vi "Set Hidden.vi"(8 "error in (no error)":errorcluster, 11 "Panel in":refnum<class "Panel.lvclass">) -> (0 "error out":errorcluster, 3 "Panel out":refnum<class "Panel.lvclass">)   [LabVIEW 2018, in "OOPanel.lvlib" / "Panel.lvclass"]
uses:
  Panel.lvclass
  State.ctl
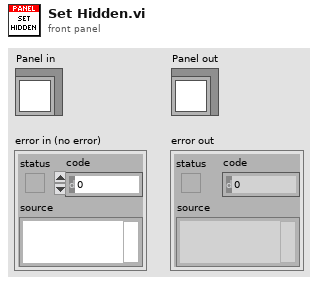
[diagram p1: front panel]
types:
  T1 = typedef "OOPanel.lvlib/Panel.lvclass/State.ctl" = enum16{"Idle", "Hidden", "Visible", "Subpanel"}
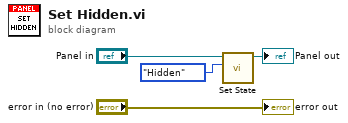
[diagram p0: block diagram]
diagram:
  n1 = call "Set State.vi"("State"=State."Hidden", "Panel in"="Panel in") -> ("Panel out"=→"Panel out":refnum<class "Panel.lvclass">)  [unwired: 8 in, 1 out]
  "error out" <- "error in (no error)"
